vi "Create SUBACK Packet.vi"(5 "SUBACK in":refnum<class "SUBACK.lvclass">, 8 "error in (no error)":errorcluster, 9 "Packet ID":u16 format="%04x", 11 "Return Codes":T1[](array[typedef])) -> (0 "error out":errorcluster, 3 "SUBACK":refnum<class "SUBACK.lvclass">)   [LabVIEW 2013, in "SUBACK.lvclass"]
uses:
  SUBACK.lvclass
  Subscription Success Code.ctl
  ControlPacket/QualityOfService -- enum.ctl
  ControlPacket/ControlPacket.lvclass/ControlPacket.ctl
  ControlPacket/ControlPacket.lvclass
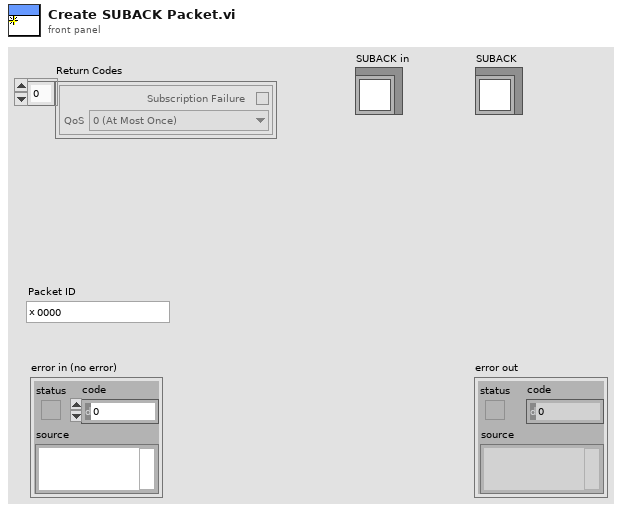
[diagram p1: front panel]
types:
  T1 = typedef "SUBACK.lvclass/Subscription Success Code.ctl" = cluster{"Subscription Failure":bool, "QoS":T2}
  T2 = typedef "ControlPacket.lvclass/QualityOfService -- enum.ctl" = enum16{"0 (At Most Once)", "1 (At Least Once)", "2 (Exactly Once)"}
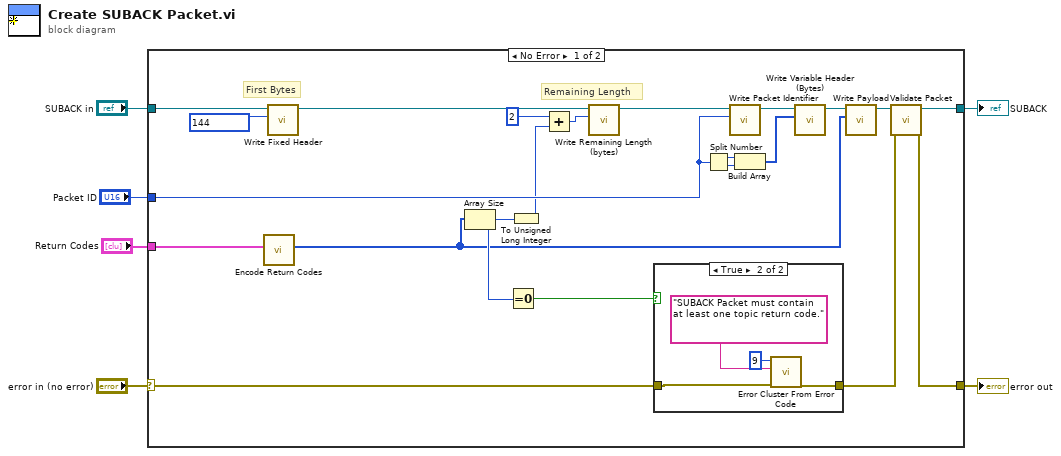
[diagram p0: block diagram]
diagram:
  n1 = case shown="No Error" "error in (no error)" {
    selector: "error in (no error)" -> [w14 w35]
    tunnel: [w7 w35] -> w3
    tunnel: [w9 w34] -> w2
    tunnel: "SUBACK in" -> [w28 w34]
    tunnel: "Packet ID" -> [w20 _]
    tunnel: "Return Codes" -> [w12 _]
    frame No Error {
      # "Remaining Length"
      # "First Bytes"
      n2 = call "Encode Return Codes.vi"("Subscription Success"=w12) -> ("Return Codes"=w11:u8[])  [unwired: 10 in]
      n3 = call "Write Fixed Header.vi"("Fixed Header"=u8 144, "ControlPacket in"=w28) -> ("ControlPacket out"=w27:refnum<class "SUBACK.lvclass">)  [unwired: 9 in]
      n4 = Array Size(array=w11) -> (size(s)=w15:i32)
      n5 = Equal To 0?(x=w15) -> (x = 0?=w13:bool)
      n6 = To Unsigned Long Integer(number=w15) -> (unsigned 32bit integer=w16:u32)
      n7 = Add(x=u32 2 ("Remaining Length (bytes)"), y=w16) -> (x+y=w18:u32)
      n8 = call "Write Remaining Length (bytes).vi"("Remaining Length (bytes)"=w18, "ControlPacket in"=w27) -> ("ControlPacket out"=w23:refnum<class "SUBACK.lvclass">)  [unwired: 9 in]
      n9 = case shown="True" w13 {
        tunnel: w14 -> [w29 w32]
        tunnel: [w29 w33] -> w8
        frame False {
        }
        frame True {
          n10 = call <vilib>:"Error Cluster From Error Code.vi"("error in (no error)"=w32, "error message (\"\")"="SUBACK Packet must contain at least one topic return code.", "error code (0)"=9) -> ("error out"=w33:errorcluster)  [unwired: 6 in]
        }
      }
      n11 = Split Number(x=w20) -> (hi(x)=w26:u8, lo(x)=w25:u8)
      n12 = call "Write Packet Identifier.vi"("Packet Identifier"=w20, "ControlPacket in"=w23) -> ("ControlPacket out"=w22:refnum<class "SUBACK.lvclass">)  [unwired: 9 in]
      n13 = Build Array(w26, w25) -> (w24:u8[])
      n14 = call "Write Variable Header (Bytes).vi"("Variable Header (Bytes)"=w24, "ControlPacket in"=w22) -> ("ControlPacket out"=w17:refnum<class "SUBACK.lvclass">)  [unwired: 9 in]
      n15 = call "Write Payload.vi"("Payload"=w11, "ControlPacket in"=w17) -> ("ControlPacket out"=w10:refnum<class "SUBACK.lvclass">)  [unwired: 9 in]
      n16 = call "Validate Packet.vi"("error in (no error)"=w8, "ControlPacket in"=w10) -> ("error out"=w7:errorcluster, "ControlPacket out"=w9:refnum<class "SUBACK.lvclass">)  [unwired: 8 in]
    }
    frame Error {
    }
  }
  "error out" <- w3
  "SUBACK" <- w2
